vi "Explore.vi"(8 "error in (no error)":errorcluster, 11 "Build Package Item in":refnum<class "VIPM Item.lvclass">) -> (0 "error out":errorcluster, 3 "Build Package Item out":refnum<class "VIPM Item.lvclass">)   [LabVIEW 2019, in "VIPM.lvlib" / "VIPM Item.lvclass"]
uses:
  VIPM Item.lvclass
  VIPM Item.lvclass/VIPM Item.ctl
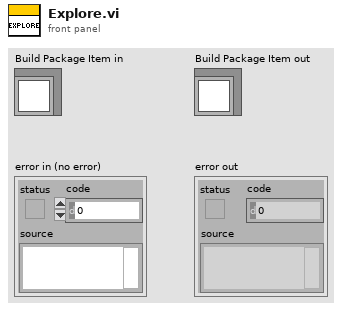
[diagram p1: front panel]
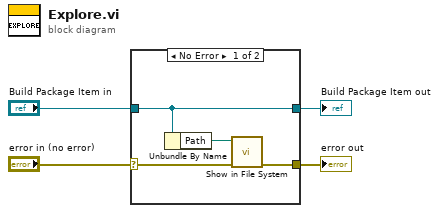
[diagram p0: block diagram]
diagram:
  n1 = case shown="No Error" "error in (no error)" {
    selector: "error in (no error)" -> [w8 w10]
    tunnel: [w7 w10] -> w3
    tunnel: [w6 w9] -> w1
    tunnel: "Build Package Item in" -> [w6 w9]
    frame No Error {
      n2 = Unbundle By Name(w6) -> ("Path"=w5:path)
      n3 = call <vilib>:"Show in File System.vi"("error in (no error)"=w8, "file or directory path"=w5) -> ("error out"=w7:errorcluster)  [unwired: 9 in]
    }
    frame Error {
    }
  }
  "error out" <- w3
  "Build Package Item out" <- w1
